vi "Initialize DMM.vi"(6 "initialize and close session behavior":T1, 8 "error in (no error)":errorcluster, 10 "reset":bool, 11 "niDMM in":refnum<class "niDMM.lvclass">) -> (0 "error out":errorcluster, 3 "niDMM out":refnum<class "niDMM.lvclass">)   [LabVIEW 2020, in "niDMM.lvclass"]
uses:
  niDMM.lvclass
  <vilib>/MeasurementLink/MeasurementLink Session Management V1/Session Reservation/Initialize and Close Session Behavior.ctl
  niDMM.lvclass/niDMM.ctl
  <vilib>/MeasurementLink/MeasurementLink niDMM/Initialize Sessions - 1Sess.vi
  <vilib>/MeasurementLink/MeasurementLink niDMM/MeasurementLink niDMM.lvlib
  <vilib>/MeasurementLink/MeasurementLink Session Management V1/Session Reservation/Session Reservation.lvclass
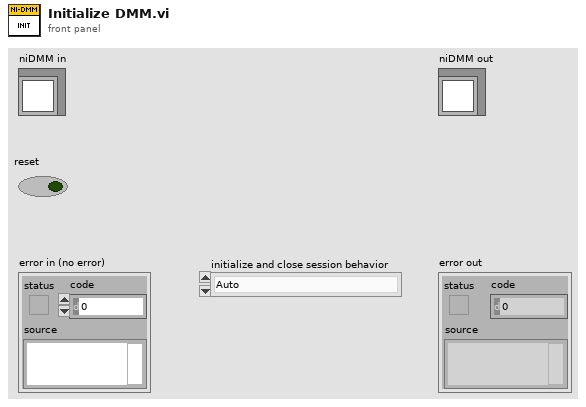
[diagram p1: front panel]
types:
  T1 = typedef "MeasurementLink Session Management V1.lvlib/Session Reservation.lvclass/Initialize and Close Session Behavior.ctl" = enum16{"Auto", "Initialize and Close", "Attach and Detach", "Initialize and Detach", "Attach and Close"}
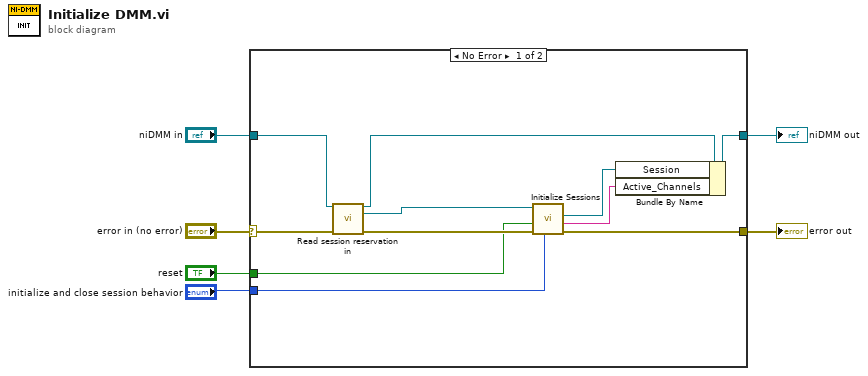
[diagram p0: block diagram]
diagram:
  n1 = case shown="No Error" "error in (no error)" {
    selector: "error in (no error)" -> [w15 w19]
    tunnel: "niDMM in" -> [w14 w18]
    tunnel: [w13 w19] -> w4
    tunnel: [w11 w18] -> w3
    tunnel: "initialize and close session behavior" -> [w8 _]
    tunnel: "reset" -> [w7 _]
    frame No Error {
      n2 = call-dynamic "Read session reservation in.vi"("AbstractDMM in"=w14, "error in (no error)"=w15) -> ("AbstractDMM out"=w12:refnum<class "niDMM.lvclass">, "MeasurementLink Session Management V1.lvlib:Session Reservation.lvclass"=w17:refnum<class "Session Reservation.lvclass">, "error out"=w16:errorcluster)  [unwired: 11 in]
      n3 = call-poly <vilib>:"Initialize Sessions.vi"("initialize and close session behavior"=w8, "error in"=w16, "reset"=w7, "session reservation in"=w17) -> ("error out"=w13:errorcluster, "channel list"=w9:string, "session"=w10:refnum<k15>)  [unwired: 4 in, 1 out]
      n4 = Bundle By Name(cluster=w12, "Session"=w10, "Active_Channels"=w9) -> (w11:refnum<class "niDMM.lvclass">)
    }
    frame Error {
    }
  }
  "error out" <- w4
  "niDMM out" <- w3
